vi "Own_Code_EV3.vi"() -> ()   [LabVIEW 2012]
uses:
  SubVIs/LVPresent_Globals.vi
  <vilib>/Platform/browser.llb/Open URL in Default Browser (string).vi
panel:
  in  "Tab Control":enum32{"Page 1", "Page 2"}(tab)
  in  "Blank Button":bool
  in  "Open":bool
  in  "Need a hint":bool
  in  "Ans. 4":bool
  in  "Ans. 3":bool
  in  "Back":bool
  # "Now it's your turn!\n\nNow that you've run through some code, let's try and write some of our own. If you are new to LabVIEW, I recommend watching the video                          .\n\nWe can start with something not too complicated like moving the car forwards for three seconds, stopping it, and then moving the car backwards the same distance.  Click the Open button to start a new VI.  Also, for now it would probably be easier to leave on AutoTooling."
  # "Step 2:\n\nAfter you get the code running and the car moving, try adding in a beeping noise when the car backs up."
  # "Check out the hints and solutions!"
  # "Hint 1: Take a look at the code from the second example. This code should be very similar, with the motor reversed when you want the device to go backwards. \n\n\n\n\n\nHint 2: To add in the beeping noise, check out the Sounds tab under the Complete, I/O, and then the MINDSTORMS Robotics tab. \n\n\n\n\n\nHelpful Tip: When creating a constant, you can simply right click on the terminal you wish to wire to, click create-->constant. Note that constants aren't always necessarily numbers."
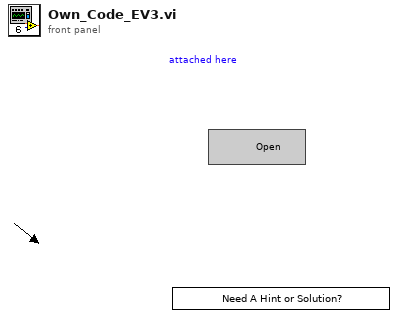
[diagram p1: front panel]
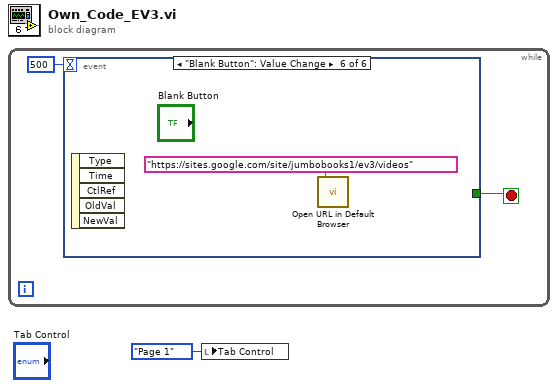
[diagram p0: block diagram]
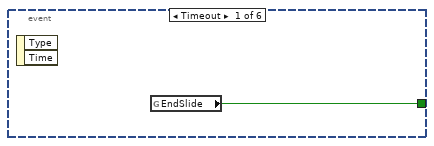
[diagram p2: hidden frame]
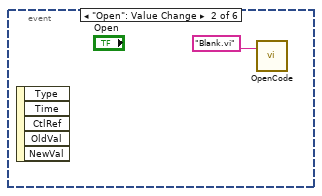
[diagram p3: hidden frame]
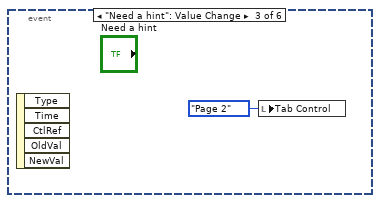
[diagram p4: hidden frame]
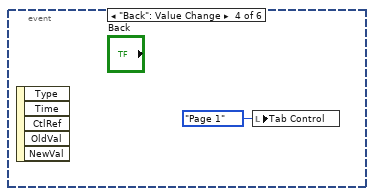
[diagram p5: hidden frame]
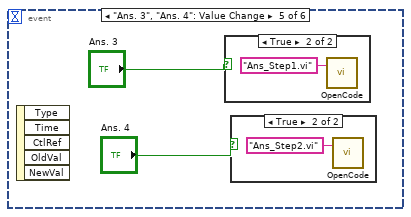
[diagram p6: hidden frame]
diagram:
  n1 = while {
    stop <- w3 stop-if-true
    n2 = event shown="[5] \"Blank Button\": Value Change" {
      selector: _ -> [_ _ _ _ _ _]
      dyn-events: _ -> [_ _ _ _ _ _]
      timeout: 500 -> [_ _ _ _ _ _]
      tunnel: [w4 _ _ _ _ _] -> w3
      event Timeout {
        n3 = event-data() -> ()  [unwired: 1 in, 2 out]
        n4 = global read "LVPresent_Globals.vi" "EndSlide"() -> (w4:bool)
      }
      event "Open": Value Change {
        n5 = event-data() -> ()  [unwired: 1 in, 5 out]
        n6 = call "OpenCode.vi"("Code name"="Blank.vi") -> ()  [unwired: 3 in]
      }
      event "Need a hint": Value Change {
        n7 = event-data() -> ()  [unwired: 1 in, 5 out]
        n8 = local write "Tab Control"(enum32{"Page 1", "Page 2"}."Page 2" ("Tab Control")) -> ()
      }
      event "Back": Value Change {
        n9 = event-data() -> ()  [unwired: 1 in, 5 out]
        n10 = local write "Tab Control"(enum32{"Page 1", "Page 2"}."Page 1" ("Tab Control")) -> ()
      }
      event "Ans. 3", "Ans. 4": Value Change {
        n11 = event-data() -> ()  [unwired: 1 in, 5 out]
        n12 = case shown="True" "Ans. 3" {
          frame False {
          }
          frame True {
            n13 = call "OpenCode.vi"("Code name"="Ans_Step1.vi") -> ()  [unwired: 3 in]
          }
        }
        n14 = case shown="True" "Ans. 4" {
          frame False {
          }
          frame True {
            n15 = call "OpenCode.vi"("Code name"="Ans_Step2.vi") -> ()  [unwired: 3 in]
          }
        }
      }
      event "Blank Button": Value Change {
        n16 = event-data() -> ()  [unwired: 1 in, 5 out]
        n17 = call-poly <vilib>:"Open URL in Default Browser.vi"("URL"="https://sites.google.com/site/jumbobooks1/ev3/videos") -> ()  [unwired: 5 in, 2 out]
      }
    }
  }
  n18 = local write "Tab Control"(enum32{"Page 1", "Page 2"}."Page 1" ("Tab Control")) -> ()
